vi "SMR_LabVIEW_V7.4.vi"() -> ()   [LabVIEW 2025]
uses:
  <vilib>/DAQmx/write.llb/DAQmx Write (Analog DBL 1Chan 1Samp).vi
  <vilib>/DAQmx/read.llb/DAQmx Read (Analog 1D DBL NChan 1Samp).vi
  <vilib>/DAQmx/create/channels.llb/DAQmx Create Channel (AI-Temperature-Thermocouple).vi
  <vilib>/DAQmx/create/channels.llb/DAQmx Create Channel (AI-Voltage-Basic).vi
  <vilib>/DAQmx/create/channels.llb/DAQmx Create Channel (AO-Voltage-Basic).vi
  <vilib>/DAQmx/miscellaneous.llb/DAQmx Fill In Error Info.vi
  <vilib>/addons/control/pid/pid.llb/PID (DBL).vi
  <vilib>/addons/control/pid/NI_PID_pid.lvlib
panel:
  out "Current Run Folder":path
  in  "Log Root Folder":path=path "C:/Users/LocalUser/Documents/GitHub/thermal-loop/resources/v0.1.1/data/001"
  out "Raw NI9201 \nVoltage Display":T1
  in  "Loop Period (ms)":dbl=1000.0
  in  "Stop":bool
  out "Auto Steady State Threshold (deg C/min)":dbl
  out "Max dT/dt (deg C/min)":dbl
  out "Temp Change Rate (deg C/min)":dbl
  out "5-Min Baseline Complete":bool
  out "Rate Window Ready":bool
  out "Steady State":bool
  in  "Voltage Limit (V)":dbl=10.0
  in  "Temperature Limit (C)":dbl=50.0
  in  "Pressure Limit (psi)":dbl=15.0
  out "Max Voltage":bool
  out "Max Temperature":bool
  out "Max Pressure":bool
  out "Heat Exchanger Pressure History":dbl(graph)
  out "Main Loop Pressure History":T2(graph)
  out "Overall Avg Pressure (psi)":dbl
  out "Heat Exchanger Pressure P6 (psi)":dbl
  out "Main Loop Avg Pressure (psi)":dbl
  out "Pressure Display":T3
  out "Overall Pressure History":T4(graph)
  out "Max Loop Pressure (psi)":dbl
  out "Heat Exchanger Temperature History":cluster{"Waveform":dbl, "Waveform":dbl}(graph)
  out "Main Loop Temeperature History":T5(graph)
  out "Heat Exchanger Avg Temp (deg C)":dbl
  out "Temperature Display":T6
  out "Overall Temperature History":T7(graph)
  out "Overall Avg Temp (deg C)":dbl
  out "Max Loop Temp (deg C)":dbl
  out "Final P-Valve Voltage (V)":dbl
  out "PID Trim Voltage (V)":dbl
  in  "PID Temp Setpoint (deg C)":dbl
  in  "Auto PID Enable":bool
  in  "Manual P-Valve Voltage (V)":dbl min=0.0 max=10.0
  out "Main Loop Avg Temp (deg C)":dbl
  in  "Flow Offset Correction (GPM)":dbl=-0.3
  out "Flow History":dbl(graph)
  out "Heat Exchanger Flow (GPM)":dbl
  # "Control/Troubleshoot"
  # "Steady State"
  # "Emergency Indicators"
  # "Pressure"
  # "Temperature"
  # "Proportional Valve Control"
  # "Heat Exchanger Flow"
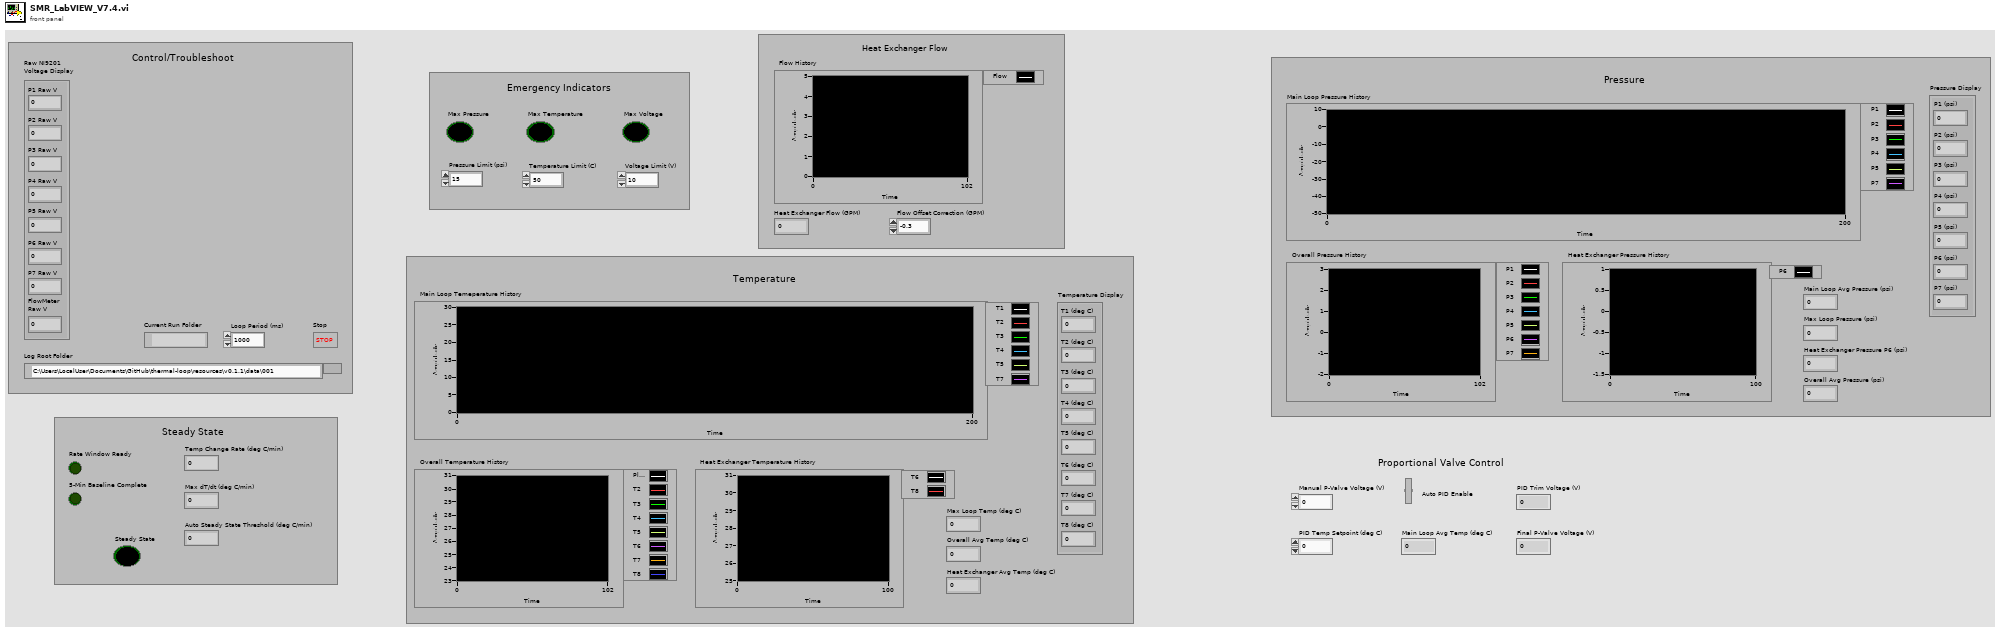
[diagram p1: front panel]
types:
  T1 = cluster{"P1 Raw V":dbl, "P2 Raw V":dbl, "P3 Raw V":dbl, "P4 Raw V":dbl, "P5 Raw V":dbl, "P6 Raw V":dbl, "P7 Raw V":dbl, "FlowMeter\nRaw V":dbl}
  T2 = cluster{"P1":dbl, "P2":dbl, "P3":dbl, "P4":dbl, "P5":dbl, "P7":dbl}
  T3 = cluster{"P1 (psi)":dbl, "P2 (psi)":dbl, "P3 (psi)":dbl, "P4 (psi)":dbl, "P5 (psi)":dbl, "P6 (psi)":dbl, "P7 (psi)":dbl}
  T4 = cluster{"P1":dbl, "P2":dbl, "P3":dbl, "P4":dbl, "P5":dbl, "P6":dbl, "P7":dbl}
  T5 = cluster{"Waveform":dbl, "Waveform":dbl, "Waveform":dbl, "Waveform":dbl, "Waveform":dbl, "Waveform":dbl}
  T6 = cluster{"T1 (deg C)":dbl, "T2 (deg C)":dbl, "T3 (deg C)":dbl, "T4 (deg C)":dbl, "T5 (deg C)":dbl, "T6 (deg C)":dbl, "T7 (deg C)":dbl, "T8 (deg C)":dbl}
  T7 = cluster{"Waveform":dbl, "Waveform":dbl, "Waveform":dbl, "Waveform":dbl, "Waveform":dbl, "Waveform":dbl, "Waveform":dbl, "Waveform":dbl}
  T8 = enum16{"open", "replace", "create", "open or create", "replace or create", "replace or create with confirmation"}
  T9 = cluster{"proportional gain (Kc)":dbl, "integral time (Ti, min)":dbl, "derivative time (Td, min)":dbl}
  T10 = cluster{"P1":dbl, "P2":dbl, "P3":dbl, "P4":dbl, "P5":dbl, "P6":dbl, "P7":dbl, "Flow":dbl}
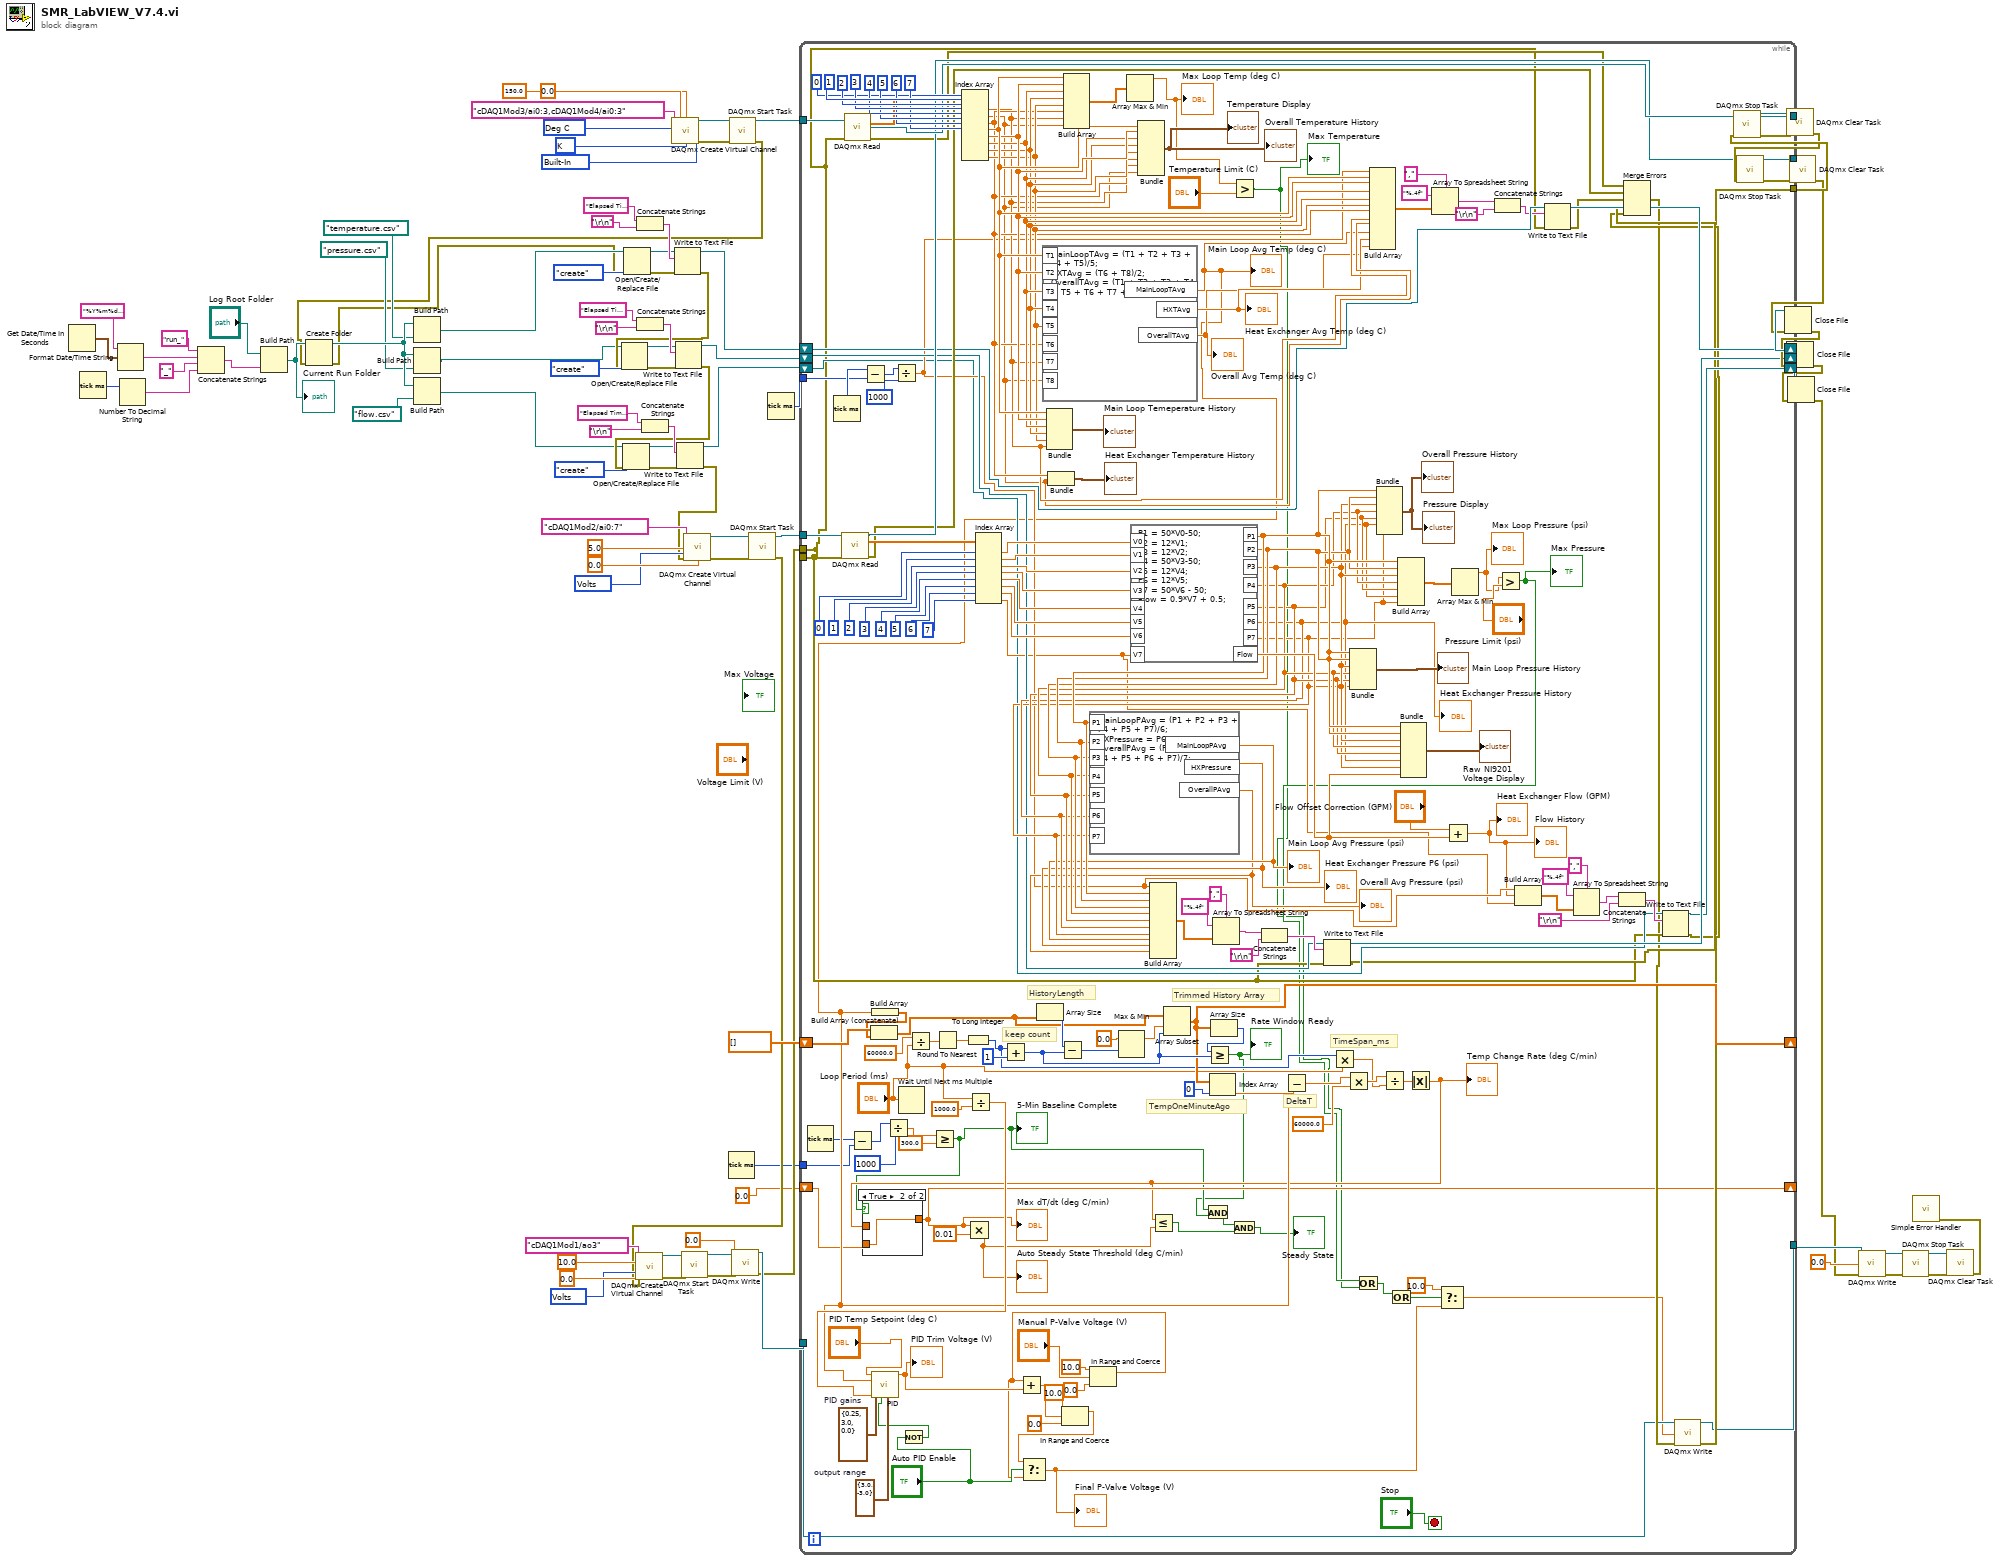
[diagram p0: block diagram]
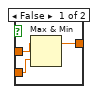
[diagram p2: hidden frame]
diagram:
  w19 = 10348 items=["Volts"=10348, "From Custom Scale"=10065] ("units")
  w85 = 10200 items=["Built-In"=10200, "Constant Value"=10116, "Channel"=10113] ("cjc source")
  w86 = 10073 items=["J"=10072, "K"=10073, "N"=10077, "R"=10082, "S"=10085, "T"=10086, "B"=10047, "E"=10055] ("thermocouple type")
  w87 = 10143 items=["Deg C"=10143, "Deg F"=10144, "Kelvins"=10325, "Deg R"=10145, "From Custom Scale"=10065] ("units")
  w94 = 10348 items=["Volts"=10348, "From Custom Scale"=10065] ("units")
  n1 = Get Date/Time In Seconds() -> (seconds since 1Jan1904=w42:timestamp)
  n2 = Tick Count (ms)() -> (millisecond timer value=w40:u32)
  n3 = Format Date/Time String(time format string (%c)="%Y%m%d_%H%M%S", seconds (now)=w42) -> (date/time string=w37:string)  [unwired: 1 in]
  n4 = Number To Decimal String(number=w40) -> (decimal integer string=w38:string)  [unwired: 1 in]
  n5 = Concatenate Strings("run_" ("string"), w37, "_" ("string"), w38) -> (w34:string)
  n6 = Build Path(base path="Log Root Folder", name or relative path=w34) -> (appended path=w33:path)
  "Current Run Folder" <- w33
  n7 = Concatenate Strings("Elapsed Time (s),T1 (deg C),T2 (deg C),T3 (deg C),T4 (deg C),T5 (deg C),T6 (deg C),T7 (deg C),T8 (deg C),Main Loop Avg Temp (deg C),HX Avg Temp (deg C),Overall Avg Temp (deg C)", "\r\n") -> (w68:string)
  n8 = Concatenate Strings("Elapsed Time (s),P1 (psi),P2 (psi),P3 (psi),P4 (psi),P5 (psi),P6 (psi),P7 (psi),Main Loop Avg Pressure (psi),HX Pressure (psi),Overall Avg Pressure (psi)", "\r\n") -> (w66:string)
  n9 = Concatenate Strings("Elapsed Time (s),Heat Exchanger Flow (GPM),Flow Raw Voltage (V)", "\r\n") -> (w62:string)
  n10 = call-poly <vilib>:"DAQmx Create Virtual Channel.vi"("maximum value"=150.0, "minimum value"=0.0, "physical channels"=tag "cDAQ1Mod3/ai0:3,cDAQ1Mod4/ai0:3", "cjc source"=w85, "units"=w87, "thermocouple type"=w86) -> ("task out"=w84:refnum<k21>, "error out"=w83:errorcluster)  [unwired: 8 in]
  n11 = Tick Count (ms)() -> (millisecond timer value=w2:u32)
  n12 = call <vilib>:"DAQmx Start Task.vi"("task/channels in"=w84, "error in"=w83) -> ("task out"=w82:refnum<k21>, "error out"=w25:errorcluster)  [unwired: 12 in]
  n13 = Create Folder(path (use dialog)=w33, error in=w25) -> (created path=w32:path, error out=w24:errorcluster)  [unwired: 1 in, 1 out]
  n14 = Build Path(base path=w32, name or relative path=path "temperature.csv") -> (appended path=w31:path)
  n15 = Build Path(base path=w32, name or relative path=path "pressure.csv") -> (appended path=w30:path)
  n16 = Build Path(base path=w32, name or relative path=path "flow.csv") -> (appended path=w29:path)
  n17 = Open/Create/Replace File(file path (use dialog)=w31, error in=w24, operation (0:open)=T8."create") -> (refnum out=w67:refnum<file>, error out=w51:errorcluster)  [unwired: 3 in, 1 out]
  n18 = Write to Text File(file (use dialog)=w67, text=w68, error in=w51) -> (refnum out=w58:refnum<file>, error out=w50:errorcluster)  [unwired: 1 in, 1 out]
  n19 = Open/Create/Replace File(file path (use dialog)=w30, error in=w50, operation (0:open)=T8."create") -> (refnum out=w65:refnum<file>, error out=w49:errorcluster)  [unwired: 3 in, 1 out]
  n20 = Write to Text File(file (use dialog)=w65, text=w66, error in=w49) -> (refnum out=w57:refnum<file>, error out=w48:errorcluster)  [unwired: 1 in, 1 out]
  n21 = Open/Create/Replace File(file path (use dialog)=w29, error in=w48, operation (0:open)=T8."create") -> (refnum out=w61:refnum<file>, error out=w47:errorcluster)  [unwired: 3 in, 1 out]
  n22 = Write to Text File(file (use dialog)=w61, text=w62, error in=w47) -> (refnum out=w56:refnum<file>, error out=w46:errorcluster)  [unwired: 1 in, 1 out]
  n23 = call-poly <vilib>:"DAQmx Create Virtual Channel.vi"("maximum value"=5.0, "minimum value"=0.0, "physical channels"=tag "cDAQ1Mod2/ai0:7", "units"=w94, "error in"=w46) -> ("task out"=w93:refnum<k21>, "error out"=w92:errorcluster)  [unwired: 9 in]
  n24 = call <vilib>:"DAQmx Start Task.vi"("task/channels in"=w93, "error in"=w92) -> ("task out"=w91:refnum<k21>, "error out"=w12:errorcluster)  [unwired: 12 in]
  n25 = call-poly <vilib>:"DAQmx Create Virtual Channel.vi"("maximum value"=10.0, "minimum value"=0.0, "physical channels"=tag "cDAQ1Mod1/ao3", "units"=w19, "error in"=w12) -> ("task out"=w18:refnum<k21>, "error out"=w17:errorcluster)  [unwired: 9 in]
  n26 = call <vilib>:"DAQmx Start Task.vi"("task/channels in"=w18, "error in"=w17) -> ("task out"=w16:refnum<k21>, "error out"=w15:errorcluster)  [unwired: 12 in]
  n27 = call-poly <vilib>:"DAQmx Write.vi"("task/channels in"=w16, "data"=0.0, "error in"=w15) -> ("task out"=w13:refnum<k21>, "error out"=w11:errorcluster)  [unwired: 10 in, 1 out]
  n28 = Tick Count (ms)() -> (millisecond timer value=w55:u32)
  n29 = while {
    tunnel: w91 -> [w263]
    tunnel: w82 -> [w237]
    tunnel: [w227] -> w81
    tunnel: [w141] -> _
    tunnel: [w226] -> w80
    tunnel: [w139] -> w79
    shift-right: [w203] -> w54
    shift-left: w58 -> [w204]
    shift-right: [w184] -> w53
    shift-left: w57 -> [w185]
    shift-right: [w173] -> w52
    shift-left: w56 -> [w174]
    tunnel: w55 -> [w222]
    shift-right: [w152] -> _
    shift-left: dbl[] [] -> [w165]
    tunnel: w13 -> [w131]
    tunnel: w11 -> [w141]
    tunnel: [w138] -> w9
    tunnel: w2 -> [w120]
    shift-right: [w113] -> _
    shift-left: 0.0 -> [w115]
    stop <- "Stop" stop-if-true
    w136 = cluster{"output high":dbl, "output low":dbl} {"output high"=3.0, "output low"=-3.0}  # output range
    w137 = T9 {"proportional gain (Kc)"=0.25, "integral time (Ti, min)"=3.0, "derivative time (Td, min)"=0.0}  # PID gains
    # "TimeSpan_ms"
    # "DeltaT"
    # "TempOneMinuteAgo"
    # "Trimmed History Array"
    # "HistoryLength"
    # "keep count"
    n30 = Tick Count (ms)() -> (millisecond timer value=w121:u32)
    n31 = Tick Count (ms)() -> (millisecond timer value=w223:u32)
    n32 = call-poly <vilib>:"DAQmx Read.vi"("task/channels in"=w263, "error in"=w141) -> ("task out"=w226:refnum<k21>, "data"=w254:dbl[], "error out"=w224:errorcluster)  [unwired: 11 in]
    n33 = call-poly <vilib>:"DAQmx Read.vi"("task/channels in"=w237, "error in"=w141) -> ("task out"=w227:refnum<k21>, "data"=w228:dbl[], "error out"=w225:errorcluster)  [unwired: 11 in]
    n34 = Subtract(x=w121, y=w120) -> (x-y=w119:u32)
    n35 = Subtract(x=w223, y=w222) -> (x-y=w221:u32)
    n36 = Divide(x=w119, y=u32 1000) -> (x/y=w117:dbl)
    n37 = Divide(x=w221, y=u32 1000) -> (x/y=w183:dbl)
    n38 = Wait Until Next ms Multiple(millisecond multiple="Loop Period (ms)") -> ()  [unwired: 1 out]
    n39 = Not(x="Auto PID Enable") -> (.not. x?=w132:bool)
    n40 = Divide(x=60000.0, y="Loop Period (ms)") -> (x/y=w162:dbl)
    n41 = Greater Or Equal?(x=w117, y=300.0) -> (x >= y?=w110:bool)
    "5-Min Baseline Complete" <- w110
    n42 = Round To Nearest(number=w162) -> (nearest integer value=w161:dbl)
    n43 = Index Array(array=w228, index #1=0 ("index"), index #2=1 ("index"), index #3=2 ("index"), index #4=3 ("index"), index #5=4 ("index"), index #6=5 ("index"), index #7=6 ("index"), index #8=7 ("index")) -> (element #1=w213:dbl, element #2=w212:dbl, element #3=w214:dbl, element #4=w219:dbl, element #5=w218:dbl, element #6=w217:dbl, element #7=w216:dbl, element #8=w215:dbl)
    n44 = To Long Integer(number=w161) -> (32bit integer=w149:i32)
    n45 = Divide(x="Loop Period (ms)", y=1000.0) -> (x/y=w133:dbl)
    n46 = Index Array(array=w254, index #1=0 ("index"), index #2=1 ("index"), index #3=2 ("index"), index #4=3 ("index"), index #5=4 ("index"), index #6=5 ("index"), index #7=6 ("index"), index #8=7 ("index")) -> (element #1=w253:dbl, element #2=w252:dbl, element #3=w251:dbl, element #4=w250:dbl, element #5=w249:dbl, element #6=w248:dbl, element #7=w247:dbl, element #8=w181:dbl)
    n47 = Add(x=w149, y=1) -> (x+y=w154:i32)
    n48 = formula code="MainLoopTAvg = (T1 + T2 + T3 + T4 + T5)/5;\nHXTAvg = (T6 + T8)/2;\nOverallTAvg = (T1 + T2 + T3 + T4 + T5 + T6 + T7 + T8)/8;"("T1"=w219, "T2"=w218, "T3"=w217, "T4"=w216, "T5"=w215, "T6"=w214, "T7"=w213, "T8"=w212) -> ("MainLoopTAvg"=w123:dbl, "HXTAvg"=w211:dbl, "OverallTAvg"=w210:dbl)
    "Overall Avg Temp (deg C)" <- w210
    "Main Loop Avg Temp (deg C)" <- w123
    "Heat Exchanger Avg Temp (deg C)" <- w211
    n49 = Build Array(w123) -> (w164:dbl[])
    n50 = Build Array (concatenate)(w165, w164) -> (w156:dbl[])
    n51 = call-poly <vilib>:"PID.vi"("reinitialize? (F)"=w132, "output range"=w136, "dt (s)"=w133, "PID gains"=w137, "process variable"=w123, "setpoint"="PID Temp Setpoint (deg C)") -> ("output"=w130:dbl)  [unwired: 4 in, 1 out]
    "PID Trim Voltage (V)" <- w130
    n52 = Array Size(array=w156) -> (size(s)=w159:i32)
    n53 = Bundle("Waveform"=w219, "Waveform"=w218, "Waveform"=w217, "Waveform"=w216, "Waveform"=w215, "Waveform"=w213) -> (→"Main Loop Temeperature History":T5)  [unwired: 1 in]
    n54 = Bundle("Waveform"=w214, "Waveform"=w212) -> (→"Heat Exchanger Temperature History":cluster{"Waveform":dbl, "Waveform":dbl})  [unwired: 1 in]
    n55 = Subtract(x=w159, y=w154) -> (x-y=w157:i32)
    n56 = Build Array(w219, w218, w217, w216, w215, w214, w213, w212) -> (w264:dbl[])
    n57 = In Range and Coerce(upper limit=10.0, x="Manual P-Valve Voltage (V)", lower limit=0.0) -> (coerced(x)=w125:dbl)  [unwired: 1 out]
    n58 = Add(x=w125, y=w130) -> (x+y=w129:dbl)
    n59 = In Range and Coerce(upper limit=10.0, x=w129, lower limit=0.0) -> (coerced(x)=w124:dbl)  [unwired: 1 out]
    n60 = Select(t=w124, s="Auto PID Enable", f=w125) -> (s? t:f=w99:dbl)
    "Final P-Valve Voltage (V)" <- w99
    n61 = Max & Min(x=0.0, y=w157) -> (max(x,y)=w155:dbl)  [unwired: 1 out]
    n62 = Array Max & Min(array=w264) -> (max value=w167:dbl)  [unwired: 3 out]
    "Max Loop Temp (deg C)" <- w167
    n63 = formula code="P1 = 50*V0-50;\nP2 = 12*V1;\nP3 = 12*V2;\nP4 = 50*V3-50;\nP5 = 12*V4;\nP6 = 12*V5; \nP7 = 50*V6 - 50;\nFlow = 0.9*V7 + 0.5;"("V0"=w253, "V1"=w252, "V2"=w251, "V3"=w250, "V4"=w249, "V5"=w248, "V6"=w247, "V7"=w181) -> ("P1"=w202:dbl, "P2"=w201:dbl, "P3"=w200:dbl, "P4"=w199:dbl, "P5"=w198:dbl, "P6"=w197:dbl, "P7"=w196:dbl, "Flow"=w242:dbl)
    "Heat Exchanger Pressure History" <- w197
    n64 = formula code="MainLoopPAvg = (P1 + P2 + P3 + P4 + P5 + P7)/6;\nHXPressure = P6;\nOverallPAvg = (P1 + P2 + P3 + P4 + P5 + P6 + P7)/7;"("P1"=w202, "P2"=w201, "P3"=w200, "P4"=w199, "P5"=w198, "P6"=w197, "P7"=w196) -> ("MainLoopPAvg"=w195:dbl, "HXPressure"=w194:dbl, "OverallPAvg"=w193:dbl)
    "Overall Avg Pressure (psi)" <- w193
    "Heat Exchanger Pressure P6 (psi)" <- w194
    "Main Loop Avg Pressure (psi)" <- w195
    n65 = Bundle("Waveform"=w219, "Waveform"=w218, "Waveform"=w217, "Waveform"=w216, "Waveform"=w215, "Waveform"=w214, "Waveform"=w213, "Waveform"=w212) -> (→"Overall Temperature History" →"Temperature Display":T7)  [unwired: 1 in]
    n66 = Build Array(w183, w202, w201, w200, w199, w198, w197, w196, w195, w194, w193) -> (w192:dbl[])
    n67 = Array Subset(array=w156, index=w155, length=w154) -> (w152:dbl[])
    n68 = Index Array(array=w152, index=0) -> (element=w150:dbl)
    n69 = Array Size(array=w152) -> (size(s)=w153:i32)
    n70 = Greater Or Equal?(x=w153, y=w154) -> (x >= y?=w109:bool)
    "Rate Window Ready" <- w109
    n71 = And(x=w110, y=w109) -> (x .and. y?=w108:bool)
    n72 = Array To Spreadsheet String(delimiter (Tab)=",", array=w192, 3:"%.4f" ("format string")) -> (spreadsheet string=w188:string)
    n73 = Greater?(x=w167, y="Temperature Limit (C)") -> (0:w104:bool)
    "Max Temperature" <- w104
    n74 = Concatenate Strings(w188, "\r\n") -> (w186:string)
    n75 = Subtract(x=w123, y=w150) -> (x-y=w148:dbl)
    n76 = Write to Text File(file (use dialog)=w185, text=w186, error in=w141) -> (refnum out=w184:refnum<file>, error out=w171:errorcluster)  [unwired: 1 in, 1 out]
    n77 = Multiply(x=w149, y="Loop Period (ms)") -> (x*y=w145:dbl)
    n78 = Multiply(x=w148, y=60000.0) -> (x*y=w146:dbl)
    n79 = Bundle("P1"=w202, "P2"=w201, "P3"=w200, "P4"=w199, "P5"=w198, "P7"=w196) -> (→"Main Loop Pressure History":T2)  [unwired: 1 in]
    n80 = Build Array(w183, w219, w218, w217, w216, w215, w214, w213, w212, w123, w211, w210) -> (w209:dbl[])
    n81 = Bundle("P1"=w202, "P2"=w201, "P3"=w200, "P4"=w199, "P5"=w198, "P6"=w197, "P7"=w196) -> (→"Overall Pressure History" →"Pressure Display":T4)  [unwired: 1 in]
    n82 = Divide(x=w146, y=w145) -> (x/y=w144:dbl)
    n83 = Build Array(w202, w201, w200, w199, w198, w197, w196) -> (w245:dbl[])
    n84 = Bundle("P1"=w202, "P2"=w201, "P3"=w200, "P4"=w199, "P5"=w198, "P6"=w197, "P7"=w196, "Flow"=w242) -> (→"Raw NI9201 \nVoltage Display":T10)  [unwired: 1 in]
    n85 = Absolute Value(x=w144) -> (abs(x)=w112:dbl)
    "Temp Change Rate (deg C/min)" <- w112
    n86 = case shown="True" w110 {
      tunnel: w115 -> [w268 w269]
      tunnel: w112 -> [w267 _]
      tunnel: [w266 w269] -> w113
      frame False {
        n87 = Max & Min(x=w267, y=w268) -> (max(x,y)=w266:dbl)  [unwired: 1 out]
      }
      frame True {
      }
    }
    "Max dT/dt (deg C/min)" <- w113
    n88 = Multiply(x=w113, y=0.01) -> (x*y=w111:dbl)
    "Auto Steady State Threshold (deg C/min)" <- w111
    n89 = Less Or Equal?(x=w112, y=w111) -> (x <= y?=w107:bool)
    n90 = And(x=w108, y=w107) -> (x .and. y?=→"Steady State":bool)
    n91 = Array To Spreadsheet String(delimiter (Tab)=",", array=w209, 3:"%.4f" ("format string")) -> (spreadsheet string=w206:string)
    n92 = Add(x="Flow Offset Correction (GPM)", y=w242) -> (x+y=w182:dbl)
    "Heat Exchanger Flow (GPM)" <- w182
    "Flow History" <- w182
    n93 = Array Max & Min(array=w245) -> (max value=w168:dbl)  [unwired: 3 out]
    "Max Loop Pressure (psi)" <- w168
    n94 = Concatenate Strings(w206, "\r\n") -> (w189:string)
    n95 = Greater?(x=w168, y="Pressure Limit (psi)") -> (0:w105:bool)
    "Max Pressure" <- w105
    n96 = Or(x=w105, y=w104) -> (x .or. y?=w103:bool)
    n97 = Or(x=w103) -> (x .or. y?=w102:bool)  [unwired: 1 in]
    n98 = Select(t=10.0, s=w102, f=w99) -> (s? t:f=w98:dbl)
    n99 = Build Array(w183, w182, w181) -> (w180:dbl[])
    n100 = Write to Text File(file (use dialog)=w204, text=w189, error in=w141) -> (refnum out=w203:refnum<file>, error out=w172:errorcluster)  [unwired: 1 in, 1 out]
    n101 = Array To Spreadsheet String(delimiter (Tab)=",", array=w180, 3:"%.4f" ("format string")) -> (spreadsheet string=w176:string)
    n102 = Concatenate Strings(w176, "\r\n") -> (w175:string)
    n103 = Write to Text File(file (use dialog)=w174, text=w175, error in=w141) -> (refnum out=w173:refnum<file>, error out=w170:errorcluster)  [unwired: 1 in, 1 out]
    n104 = Merge Errors(w225, w224, w172, w171, w170) -> (w140:errorcluster)
    n105 = call-poly <vilib>:"DAQmx Write.vi"("task/channels in"=w131, "data"=w98, "error in"=w140) -> ("task out"=w138:refnum<k21>, "error out"=w139:errorcluster)  [unwired: 10 in, 1 out]
  }
  n106 = call <vilib>:"DAQmx Stop Task.vi"("task/channels in"=w81, "error in"=w79) -> ("task out"=w78:refnum<k21>, "error out"=w76:errorcluster)  [unwired: 12 in]
  n107 = call <vilib>:"DAQmx Clear Task.vi"("task in"=w78, "error in"=w76) -> ("error out"=w75:errorcluster)  [unwired: 13 in]
  n108 = call <vilib>:"DAQmx Stop Task.vi"("task/channels in"=w80, "error in"=w75) -> ("task out"=w77:refnum<k21>, "error out"=w74:errorcluster)  [unwired: 12 in]
  n109 = call <vilib>:"DAQmx Clear Task.vi"("task in"=w77, "error in"=w74) -> ("error out"=w45:errorcluster)  [unwired: 13 in]
  n110 = Close File(refnum=w54, error in=w45) -> (error out=w44:errorcluster)  [unwired: 1 out]
  n111 = Close File(refnum=w53, error in=w44) -> (error out=w43:errorcluster)  [unwired: 1 out]
  n112 = Close File(refnum=w52, error in=w43) -> (error out=w8:errorcluster)  [unwired: 1 out]
  n113 = call-poly <vilib>:"DAQmx Write.vi"("task/channels in"=w9, "data"=0.0, "error in"=w8) -> ("task out"=w7:refnum<k21>, "error out"=w5:errorcluster)  [unwired: 10 in, 1 out]
  n114 = call <vilib>:"DAQmx Stop Task.vi"("task/channels in"=w7, "error in"=w5) -> ("task out"=w6:refnum<k21>, "error out"=w4:errorcluster)  [unwired: 12 in]
  n115 = call <vilib>:"DAQmx Clear Task.vi"("task in"=w6, "error in"=w4) -> ("error out"=w3:errorcluster)  [unwired: 13 in]
  n116 = call <vilib>:"Simple Error Handler.vi"("error in (no error)"=w3) -> ()  [unwired: 4 in, 5 out]
